vi "Data_Bios.vi"(7 "error in (no error)":errorcluster) -> (0 "error out":errorcluster, 1 "Hora":string, 3 "Data":string)   [LabVIEW 2019]
panel:
  # "sync clock to NIST time"
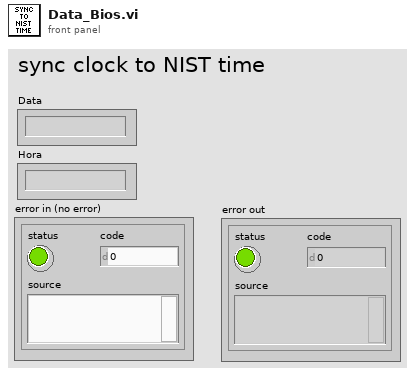
[diagram p1: front panel]
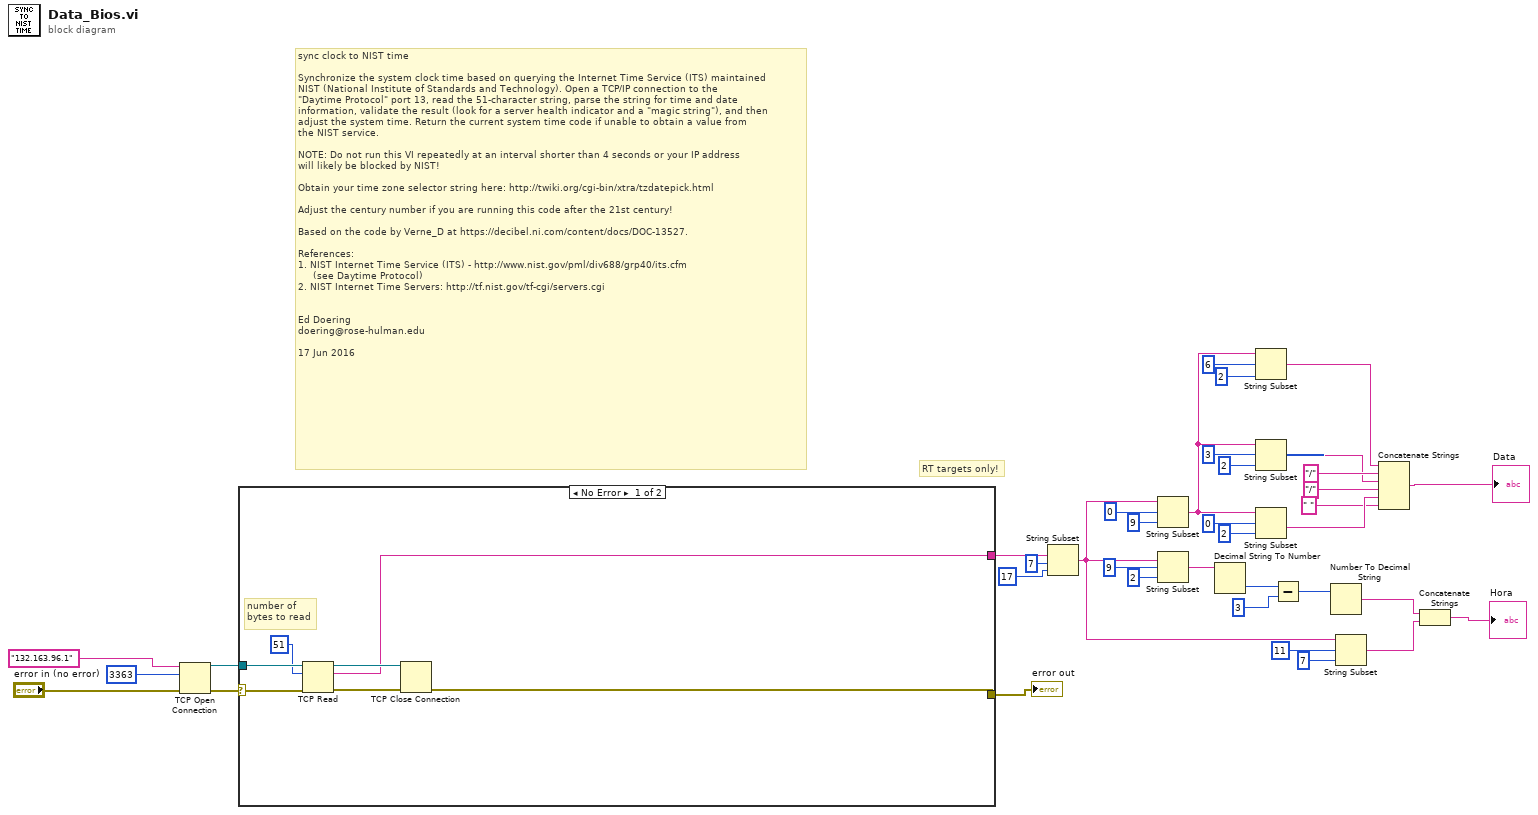
[diagram p0: block diagram]
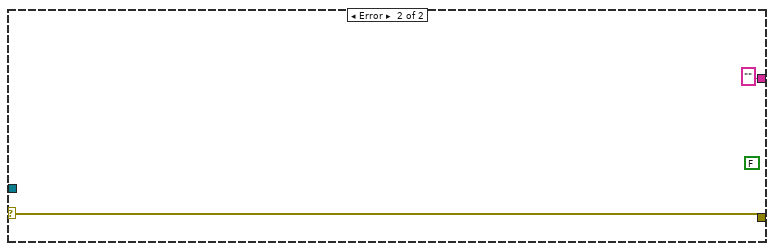
[diagram p2: hidden frame]
diagram:
  # "RT targets only!"
  # "sync clock to NIST time\n\nSynchronize the system clock time based on querying the Internet Time Service (ITS) maintained\nNIST (National Institute of Standards and Technology). Open a TCP/IP connection to the\n\"Daytime Protocol\" port 13, read the 51-character string, parse the string for time and date \ninformation, validate the result (look for a server health indicator and a \"magic string\"), and then\nadjust the system time. Return the current system time code if unable to obtain a value from\nthe NIST service.\n\nNOTE: Do not run this VI repeatedly at an interval shorter than 4 seconds or your IP address\nwill likely be blocked by NIST!\n\nObtain your time zone selector string here: http://twiki.org/cgi-bin/xtra/tzdatepick.html \n\nAdjust the century number if you are running this code after the 21st century!\n\nBased on the code by Verne_D at https://decibel.ni.com/content/docs/DOC-13527.\n\nReferences:\n1. NIST Internet Time Service (ITS) - http://www.nist.gov/pml/div688/grp40/its.cfm\n     (see Daytime Protocol) \n2. NIST Internet Time Servers: http://tf.nist.gov/tf-cgi/servers.cgi \n\n\nEd Doering\ndoering@rose-hulman.edu\n\n17 Jun 2016"
  n1 = TCP Open Connection(address="132.163.96.1" ("NIST time server IP address"), remote port or service name=u16 3363 ("port"), error in (no error)="error in (no error)") -> (connection ID=w34:refnum<k5>, error out=w35:errorcluster)  [unwired: 2 in]
  n2 = case shown="No Error" w35 {
    selector: w35 -> [w44 w45]
    tunnel: w34 -> [w43 _]
    tunnel: [w38 w45] -> w33
    tunnel: [w40 "" ("data out")] -> w31
    frame No Error {
      # "number of\nbytes to read"
      n3 = TCP Read(connection ID=w43, bytes to read=51, error in (no error)=w44) -> (connection ID out=w41:refnum<k5>, data out=w40:string, error out=w42:errorcluster)  [unwired: 2 in]
      n4 = TCP Close Connection(connection ID=w41, error in (no error)=w42) -> (error out=w38:errorcluster)  [unwired: 1 in, 1 out]
    }
    frame Error {
      (unwired) FALSE
    }
  }
  "error out" <- w33
  n5 = String Subset(string=w31, offset (0)=7, length (rest)=17 ("length (rest)")) -> (substring=w21:string)
  n6 = String Subset(string=w21, offset (0)=0, length (rest)=9 ("length (rest)")) -> (substring=w14:string)
  n7 = String Subset(string=w21, offset (0)=9, length (rest)=2 ("length (rest)")) -> (substring=w27:string)
  n8 = Decimal String To Number(string=w27) -> (number=w26:i32)  [unwired: 2 in, 1 out]
  n9 = String Subset(string=w14, offset (0)=6, length (rest)=2 ("length (rest)")) -> (substring=w11:string)
  n10 = String Subset(string=w14, offset (0)=3, length (rest)=2 ("length (rest)")) -> (substring=w9:string)
  n11 = String Subset(string=w14, offset (0)=0, length (rest)=2 ("length (rest)")) -> (substring=w7:string)
  n12 = Subtract(x=w26, y=3) -> (x-y=w22:i32)
  n13 = Number To Decimal String(number=w22) -> (decimal integer string=w3:string)  [unwired: 1 in]
  n14 = String Subset(string=w21, offset (0)=11, length (rest)=7 ("length (rest)")) -> (substring=w4:string)
  n15 = Concatenate Strings(w11, "/" ("string"), w9, "/" ("string"), w7, " " ("string")) -> (→"Data":string)
  n16 = Concatenate Strings(w3, w4) -> (→"Hora":string)
